vi "未命名 1.vi"() -> ()   [LabVIEW 2013]
uses:
  InitConfig.ctl
panel:
  in  "Transmit Channel":u32(ring) items=["0", "1"]
  in  "ID(Hex 高位有效)":string="80 00 00 00" caption="ff"
  in  "Data Input(Hex)":string="11 22 33 44 55 66 77 88"
  in  "Frame Format":u8(ring) items=["Data Frame", "Remote Frame"]
  in  "Frame Type":u8(ring) items=["Standard Frame", "Extend Frame"]
  in  "Transmit Type":u8(ring) items=["Normal Transmit"]
  in  "CanRx_IER":u8(ring)=1 items=["0", "1"]
  in  "kCanBaud":u8(ring)=10 items=["250k bps"=10, "10k bps"=2, "5k bps"=1, "50k bps"=5, "40k bps"=4, "20k bps"=3, "80k bps"=6, "100k bps"=7, "125k bps"=8, "200k bps"=9, "400k bps"=11, "500k bps"=12, "666k bps"=13, "800k bps"=14, "1000k bps"=15]
  in  "Mode":u8(ring) items=["Normal", "Self TX-RX"]
  in  "Filter":u8(ring) items=["Single Filter", "Dual Filter"]
  in  "AccCode":u32 format="0x%08x"
  in  "AccMask":u32=4294967295 format="0x%08x"
  out "Result 5":bool=TRUE
  out "Result 4":bool
  out "Result 3":bool=TRUE
  out "Result 2":bool=TRUE
  out "Result":bool=TRUE
  out "ReceiveData":T1 {"?" format="%x"; "?" format="%x"; "?" format="%x"; "?" format="%x"; "?" format="%x"; "?" format="%x"; "?" format="%x"; "?" format="%x"; "ID" format="%x"}
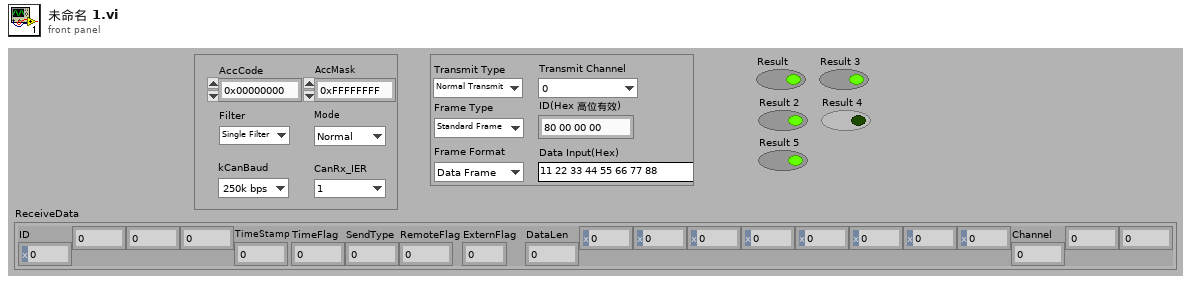
[diagram p1: front panel]
types:
  T1 = cluster{"ID":u8, u8, u8, u8, "TimeStamp":u32, "TimeFlag":u8, "SendType":u8, "RemoteFlag":u8, "ExternFlag":u8, "DataLen":u8, u8, u8, u8, u8, u8, u8, u8, u8, "Channel":u8, u8, u8}
  T2 = cluster{"Transmit Type":u8, "Frame Type":u8, "Frame Format":u8, "Data Input(Hex)":string, "ID(Hex 高位有效)":string}
  T3 = typedef "InitConfig.ctl" = cluster{"AccCode":u32, "AccMask":u32, "Reserved":u32, "Filter":u8, "kCanBaud":u8, "Timing0":u8, "Timing1":u8, "Mode":u8, "CanRx_IER":u8}
  T4 = cluster{"ID":u8, u8, u8, u8, "TimeStamp":u32, "TimeFlag":u8, "SendType":u8, "RemoteFlag":u8, "ExternFlag":u8, "DataLen":u8, "Byte0":u8, "Byte1":u8, "Byte2":u8, "Byte3":u8, "Byte4":u8, "Byte5":u8, "Byte6":u8, "Byte7":u8, "Channel":u8, u8, u8}
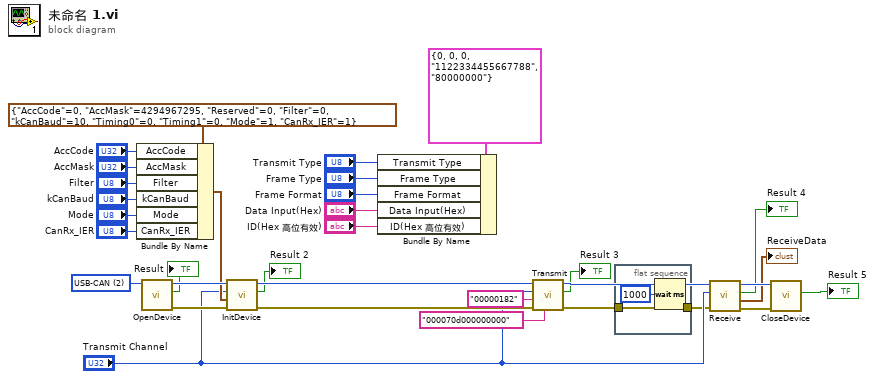
[diagram p0: block diagram]
diagram:
  w26 = u16 2 items=["PCI-CAN200"=7, "USB-CAN"=2] ("DeviceType")
  n1 = Bundle By Name(cluster=T3 {"AccCode"=0, "AccMask"=4294967295, "Reserved"=0, "Filter"=0, "kCanBaud"=10, "Timing0"=0, "Timing1"=0, "Mode"=1, "CanRx_IER"=1} ("pInitConfig"), "AccCode"="AccCode", "AccMask"="AccMask", "Filter"="Filter", "kCanBaud"="kCanBaud", "Mode"="Mode", "CanRx_IER"="CanRx_IER") -> (w18:T3)
  n2 = call "OpenDevice.vi"("DeviceType"=w26) -> ("错误输出"=w29:errorcluster, "Result"=→"Result":bool, "DeviceTypeOut"=w33:u16)  [unwired: 8 in]
  n3 = call "InitDevice.vi"("错误输入（无错误）"=w29, "InitConfig"=w18, "CanChannel"="Transmit Channel", "DeviceType"=w33) -> ("错误输出"=w28:errorcluster, "Result"=→"Result 2":bool, "DeviceTypeOut"=w32:u16)  [unwired: 5 in]
  n4 = Bundle By Name(cluster=T2 {"Transmit Type"=0, "Frame Type"=0, "Frame Format"=0, "Data Input(Hex)"="1122334455667788", "ID(Hex 高位有效)"="80000000"} ("CanParas"), "Transmit Type"="Transmit Type", "Frame Type"="Frame Type", "Frame Format"="Frame Format", "Data Input(Hex)"="Data Input(Hex)", "ID(Hex 高位有效)"="ID(Hex 高位有效)") -> ()  [unwired: 1 out]
  n5 = call "Transmit.vi"("Data Input(Hex)"="000070d000000000", "错误输入（无错误）"=w28, "ID(Hex 高位有效)"="00000182", "CANChannel"="Transmit Channel", "DeviceType"=w32) -> ("错误输出"=w4:errorcluster, "Result"=→"Result 3":bool, "DeviceTypeOut"=w31:u16)  [unwired: 4 in]
  n6 = flat-sequence {
    tunnel: w4 -> [w35]
    tunnel: [w35] -> w3
    frame #0 {
      n7 = Wait (ms)(milliseconds to wait=u32 1000 ("等待时间（毫秒）")) -> ()  [unwired: 1 out]
    }
  }
  n8 = call "Receive.vi"("错误输入（无错误）"=w3, "CANChannel"="Transmit Channel", "DeviceType"=w31) -> ("错误输出"=w27:errorcluster, "VCI_CAN_OBJ_R"=→"ReceiveData":T4, "Result"=→"Result 4":bool, "DeviceTypeOut"=w30:u16)  [unwired: 5 in]
  n9 = call "CloseDevice.vi"("错误输入（无错误）"=w27, "DeviceType"=w30) -> ("Result"=→"Result 5":bool)  [unwired: 7 in, 2 out]
